vi "Create.vi"(8 "error in (no error)":errorcluster, 10 "Input":string[](array[string])) -> (0 "error out":errorcluster, 3 "Range Map":refnum<class "Range Map.lvclass">)   [LabVIEW 2020, in "Range Map.lvclass"]
uses:
  Range Map.lvclass
  Range/Range.lvclass
  Range Map.lvclass/Range Map.ctl
  Map/Map.lvclass
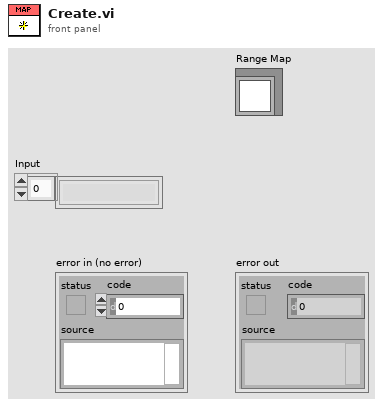
[diagram p1: front panel]
types:
  T1 = cluster{"Source":refnum<class "Range.lvclass">, "Destination":refnum<class "Range.lvclass">}
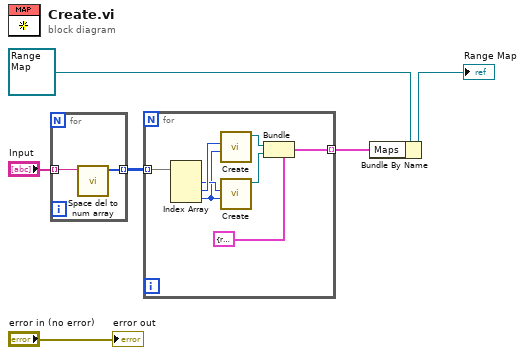
[diagram p0: block diagram]
diagram:
  n1 = for {
    tunnel: "Input" -> [w8] mode=indexing
    tunnel: [w7] -> w3 mode=indexing
    n2 = call "Space del to num array.vi"("Input in"=w8) -> ("Input out"=w7:u64[])  [unwired: 10 in]
  }
  n3 = for {
    tunnel: w3 -> [w16] mode=indexing
    tunnel: [w9] -> w1 mode=indexing
    n4 = Index Array(array=w16) -> (element #1=w13:u64, element #2=w15:u64, element #3=w12:u64)  [unwired: 3 in]
    n5 = call "Create.vi"("Length"=w12, "From"=w15) -> ("Range"=w14:refnum<class "Range.lvclass">)  [unwired: 8 in, 1 out]
    n6 = call "Create.vi"("Length"=w12, "From"=w13) -> ("Range"=w11:refnum<class "Range.lvclass">)  [unwired: 8 in, 1 out]
    n7 = Bundle(cluster=T1 {"Source"=refnum, "Destination"=refnum}, "Source"=w14, "Destination"=w11) -> (w9:T1)
  }
  n8 = Bundle By Name(cluster=refnum<class "Range Map.lvclass"> refnum ("Range Map"), "Maps"=w1) -> (→"Range Map":refnum<class "Range Map.lvclass">)
  "error out" <- "error in (no error)"
